vi "VsEPCal-Set Atten.vi"(0 "Runtime":T1, 11 "error in (no error)":errorcluster) -> (4 "Runtime out":T1, 14 "Level":dbl, 15 "error out":errorcluster)   [LabVIEW 2020]
uses:
  Typedefs/VsEP-Runtime Data.ctl
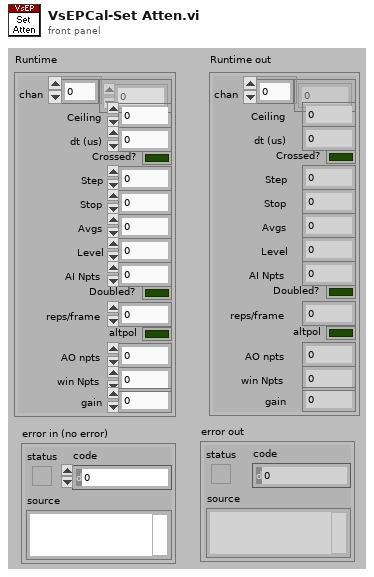
[diagram p1: front panel]
types:
  T1 = typedef "VsEP-Runtime Data.ctl" = cluster{"chan":i32[], "Ceiling":dbl, "dt (us)":dbl, "Crossed?":bool, "Step":dbl, "Stop":i32, "Avgs":i32, "Level":dbl, "AI Npts":i32, "Doubled?":bool, "reps/frame":i32, "altpol":bool, "AO npts":i32, "win Npts":i32, "gain":dbl}
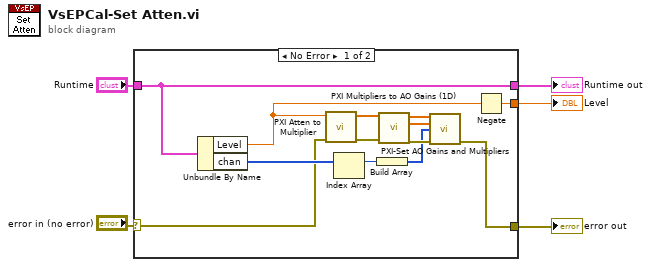
[diagram p0: block diagram]
diagram:
  n1 = case shown="No Error" "error in (no error)" {
    selector: "error in (no error)" -> [w11 w19]
    tunnel: "Runtime" -> [w9 w20]
    tunnel: [w9 w20] -> w3
    tunnel: [w10 w19] -> w2
    tunnel: [w7 _] -> w1
    frame No Error {
      n2 = Unbundle By Name(w9) -> ("Level"=w8:dbl, "chan"=w13:i32[])
      n3 = call "PXI Atten to Multiplier.vi"("error in (no error)"=w11, "Attenuation"=w8) -> ("error out"=w17:errorcluster, "Multiplier setting"=w18:dbl[])  [unwired: 8 in]
      n4 = Index Array(array=w13) -> (element=w6:i32)  [unwired: 1 in]
      n5 = Build Array(w6) -> (w12:i32[])
      n6 = call "PXI Multipliers to AO Gains (1D).vi"("Multipliers in"=w18, "error in (no error)"=w17) -> ("Multipliers out"=w14:dbl[], "Gains"=w15:dbl[], "error out"=w16:errorcluster)  [unwired: 11 in]
      n7 = call "PXI-Set AO Gains and Multipliers.vi"("Multipliers"=w14, "Gains"=w15, "AO Channels"=w12, "error in (no error)"=w16) -> ("error out"=w10:errorcluster)  [unwired: 11 in]
      n8 = Negate(x=w8) -> (-x=w7:dbl)
    }
    frame Error {
    }
  }
  "error out" <- w2
  "Level" <- w1
  "Runtime out" <- w3
